vi "Parse Sequence Command.vi"(0 "Current Test":string[](array[string])) -> (1 "error out":errorcluster, 2 "input cluster":T1)   [LabVIEW 2010]
uses:
  Sequence Table Cluster TDef.ctl
panel:
  in  "Index of Actual Column":i32=2
  in  "Test Table 2":string[][](array[string])=[["1", "10mA", "1", "", ""], ["2", "1", "2", "", ""], ["3", "100mA", "1", "[1]+175", ""], ["4", "20mA", "4", "", ""]]
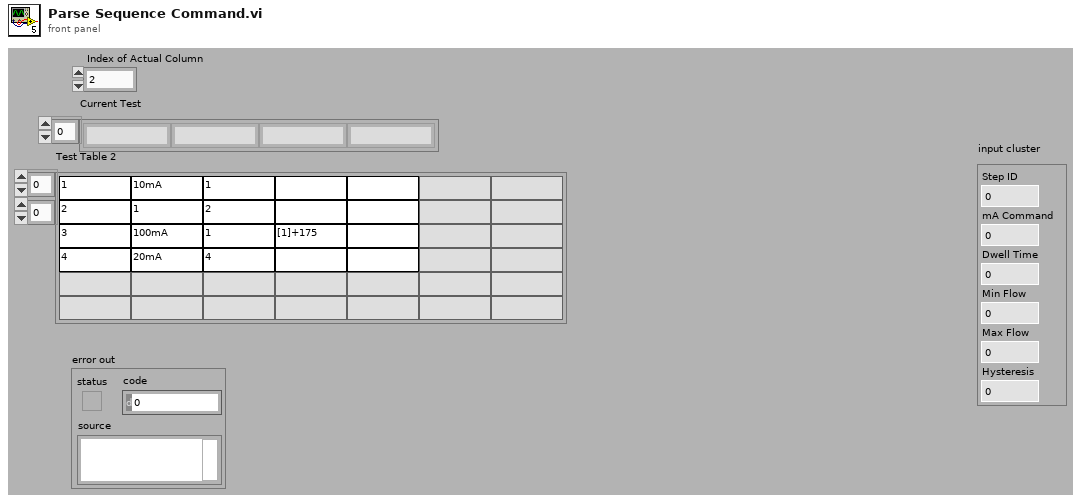
[diagram p1: front panel]
types:
  T1 = typedef "Sequence Table Cluster TDef.ctl" = cluster{"Step ID":i32, "mA Command":dbl, "Dwell Time":dbl, "Min Flow":dbl, "Max Flow":dbl, "Hysteresis":dbl}
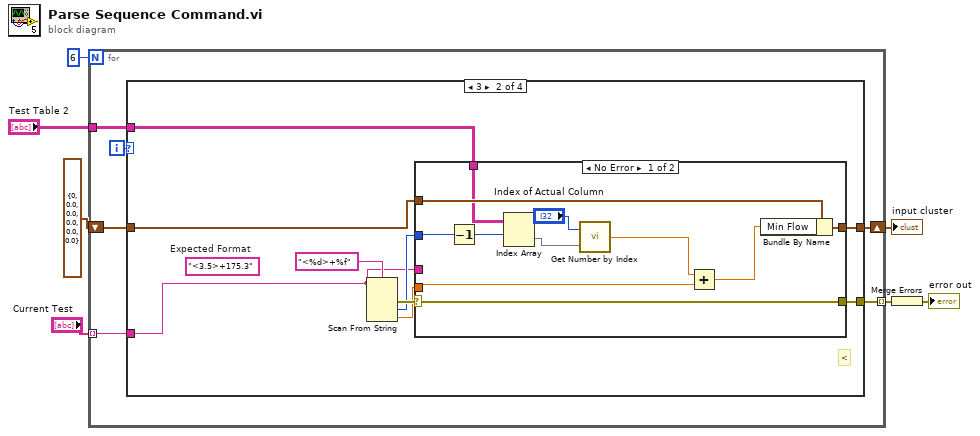
[diagram p0: block diagram]
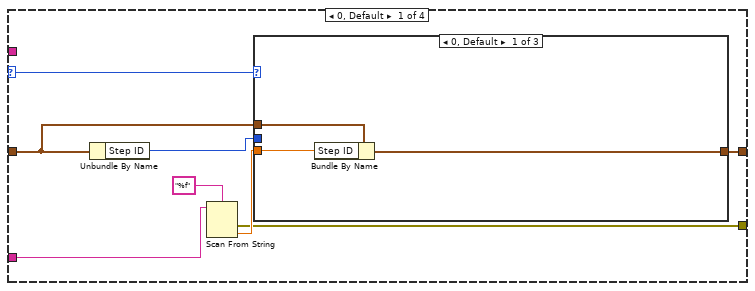
[diagram p2: hidden frame]
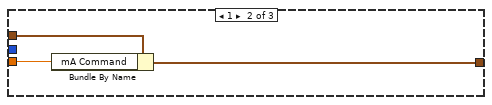
[diagram p3: hidden frame]
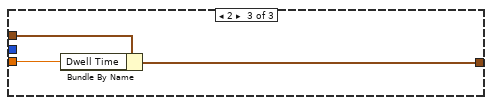
[diagram p4: hidden frame]
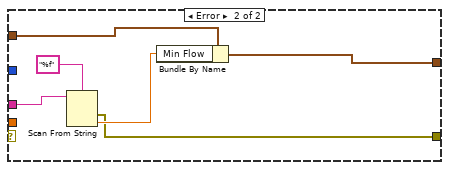
[diagram p5: hidden frame]
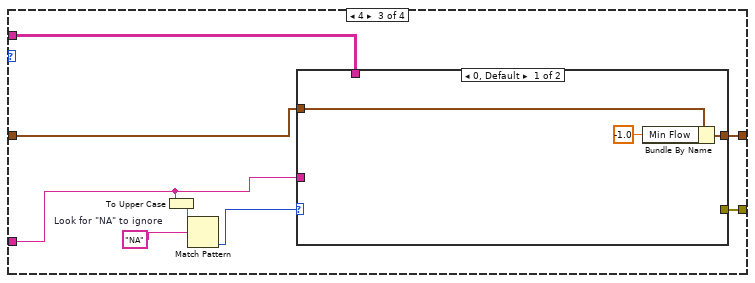
[diagram p6: hidden frame]
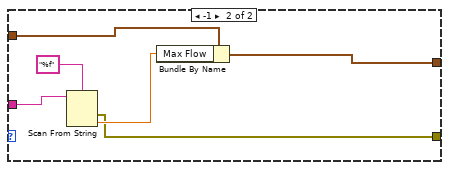
[diagram p7: hidden frame]
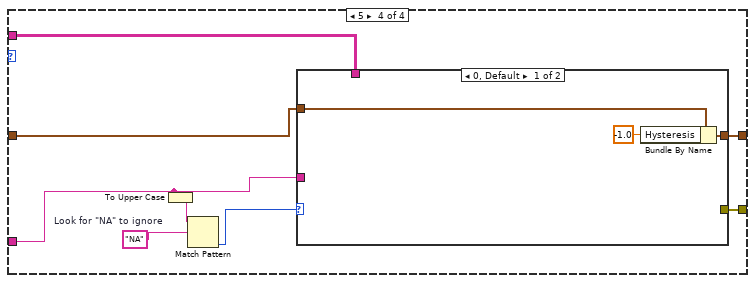
[diagram p8: hidden frame]
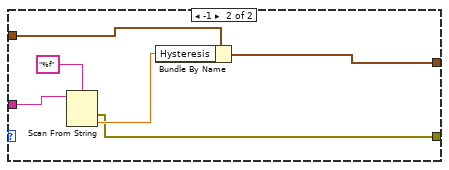
[diagram p9: hidden frame]
diagram:
  n1 = for {
    N: 6 -> [_]
    tunnel: "Current Test" -> [w12] mode=indexing
    tunnel: [w11] -> w6 mode=indexing
    shift-right: [w9] -> w5
    shift-left: T1 {"Step ID"=0, "mA Command"=0.0, "Dwell Time"=0.0, "Min Flow"=0.0, "Max Flow"=0.0, "Hysteresis"=0.0} ("input cluster") -> [w10]
    tunnel: "Test Table 2" -> [w8]
    i -> [w13]
    n2 = case shown="3" w13 {
      selector: w13 -> [w19 _ _ _]
      tunnel: w12 -> [w20 w31 w60 w77]
      tunnel: [w14 w37 w58 w75] -> w11
      tunnel: w10 -> [w16 w36 w64 w81]
      tunnel: [w18 w35 w63 w80] -> w9
      tunnel: w8 -> [_ w32 w62 w79]
      frame 0, Default {
        n3 = Unbundle By Name(w16) -> ("Step ID"=w15:i32)
        n4 = Scan From String(format string="%f", input string=w20) -> (error out=w14:errorcluster, output 1=w17:dbl)  [unwired: 3 in, 2 out]
        n5 = case shown="0, Default" w19 {
          tunnel: w16 -> [w24 w27 w30]
          tunnel: [w23 w26 w29] -> w18
          tunnel: w17 -> [w22 w25 w28]
          tunnel: w15 -> [_ _ _]
          frame 0, Default {
            n6 = Bundle By Name(cluster=w24, "Step ID"=w22) -> (w23:T1)
          }
          frame 1 {
            n7 = Bundle By Name(cluster=w27, "mA Command"=w25) -> (w26:T1)
          }
          frame 2 {
            n8 = Bundle By Name(cluster=w30, "Dwell Time"=w28) -> (w29:T1)
          }
        }
      }
      frame 3 {
        (unwired) "<3.5>+175.3"  # Expected Format
        # "<"
        n9 = Scan From String(format string="<%d>+%f", input string=w31) -> (error out=w38:errorcluster, output 1=w34:i32, output 2=w33:dbl)  [unwired: 4 in, 2 out]
        n10 = case shown="No Error" w38 {
          selector: w38 -> [w50 _]
          tunnel: [w50 w51] -> w37
          tunnel: w36 -> [w49 w56]
          tunnel: [w48 w55] -> w35
          tunnel: w34 -> [w46 _]
          tunnel: w33 -> [w41 _]
          tunnel: w32 -> [w47 _]
          tunnel: w31 -> [_ w54]
          frame No Error {
            n11 = Decrement(x=w46) -> (x-1=w45:i32)
            n12 = Index Array(array=w47, index (row)=w45) -> (element=w44:string[])  [unwired: 1 in]
            n13 = call "Get Number by Index.vi"("Test Table"=w44, "Index"="Index of Actual Column") -> ("Dwell Time"=w42:dbl)
            n14 = Add(x=w42, y=w41) -> (x+y=w40:dbl)
            n15 = Bundle By Name(cluster=w49, "Min Flow"=w40) -> (w48:T1)
          }
          frame Error {
            n16 = Scan From String(format string="%f", input string=w54) -> (error out=w51:errorcluster, output 1=w52:dbl)  [unwired: 3 in, 2 out]
            n17 = Bundle By Name(cluster=w56, "Min Flow"=w52) -> (w55:T1)
          }
        }
      }
      frame 4 {
        w61 = "NA"  # Look for "NA" to ignore
        n18 = To Upper Case(1:w60) -> (0:w57:string)
        n19 = Match Pattern(string=w57, regular expression=w61) -> (offset past match=w59:i32)  [unwired: 1 in, 3 out]
        n20 = case shown="0, Default" w59 {
          tunnel: [_ w68] -> w58
          tunnel: w64 -> [w67 w73]
          tunnel: [w66 w72] -> w63
          tunnel: w62 -> [_ _]
          tunnel: w60 -> [_ w71]
          frame 0, Default {
            n21 = Bundle By Name(cluster=w67, "Min Flow"=-1.0) -> (w66:T1)
          }
          frame -1 {
            n22 = Scan From String(format string="%f", input string=w71) -> (error out=w68:errorcluster, output 1=w69:dbl)  [unwired: 3 in, 2 out]
            n23 = Bundle By Name(cluster=w73, "Max Flow"=w69) -> (w72:T1)
          }
        }
      }
      frame 5 {
        w78 = "NA"  # Look for "NA" to ignore
        n24 = To Upper Case(1:w77) -> (0:w74:string)
        n25 = Match Pattern(string=w74, regular expression=w78) -> (offset past match=w76:i32)  [unwired: 1 in, 3 out]
        n26 = case shown="0, Default" w76 {
          tunnel: w81 -> [w84 w90]
          tunnel: [w83 w89] -> w80
          tunnel: w79 -> [_ _]
          tunnel: w77 -> [_ w88]
          tunnel: [_ w85] -> w75
          frame 0, Default {
            n27 = Bundle By Name(cluster=w84, "Hysteresis"=-1.0 ("Min Flow")) -> (w83:T1)
          }
          frame -1 {
            n28 = Scan From String(format string="%f", input string=w88) -> (error out=w85:errorcluster, output 1=w86:dbl)  [unwired: 3 in, 2 out]
            n29 = Bundle By Name(cluster=w90, "Hysteresis"=w86) -> (w89:T1)
          }
        }
      }
    }
  }
  "input cluster" <- w5
  n30 = Merge Errors(w6) -> (→"error out":errorcluster)
